vi "CAP-MOD-4.vi"(0 "Count per volt":dbl, 1 "Boolean 3":bool, 2 "Numeric 10":dbl, 3 "data[2]":u8, 4 "data[3]":u8, 5 "data[4]":u8, 6 "data[5]":u8, 8 "Boolean":bool, 9 "data[6]":u8, 10 "Boolean 2":bool, 11 "data[7]":u8, 12 "Numeric 9":dbl, 13 "Numeric 12":dbl, 14 "Numeric 8":dbl, 15 "Numeric 11":dbl, 16 "Numeric 7":dbl) -> (18 "Numeric 4":dbl, 20 "Numeric 5":dbl, 21 "Numeric 6":dbl, 22 "Numeric 3":dbl, 23 "Numeric":dbl, 24 "Numeric 2":dbl)   [LabVIEW 2016]
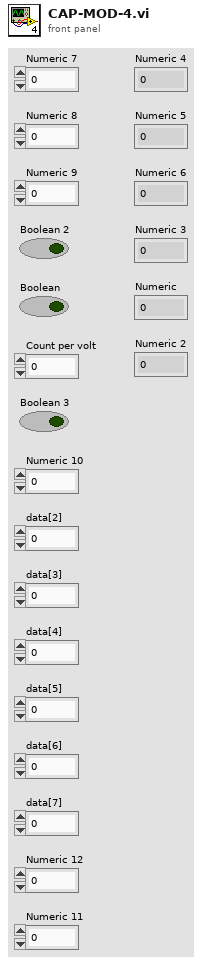
[diagram p1: front panel]
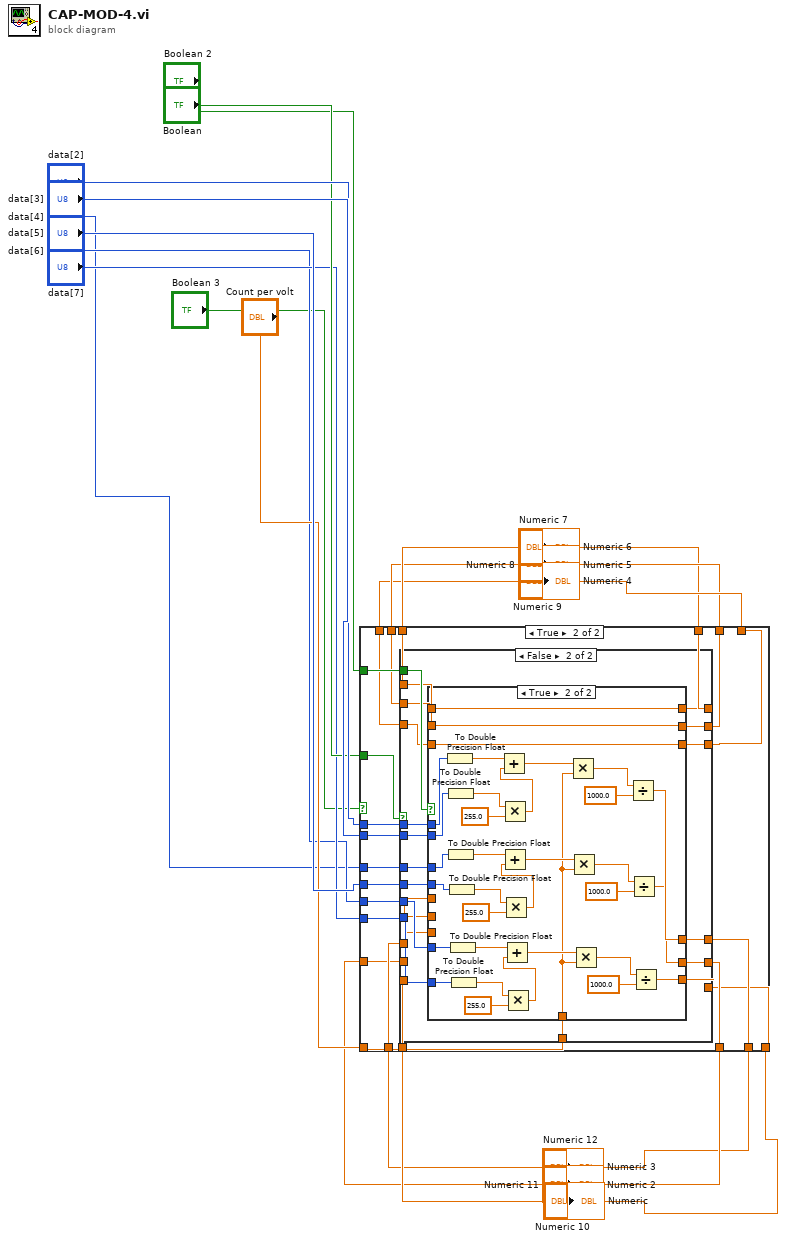
[diagram p0: block diagram]
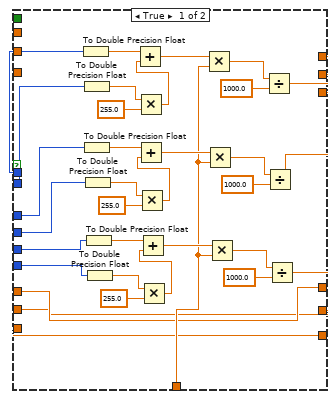
[diagram p3: hidden frame]
diagram:
  n1 = case shown="True" "Boolean 3" {
    tunnel: "Boolean 2" -> [_ w49]
    tunnel: "Boolean" -> [_ w48]
    tunnel: [w23 w47] -> w15
    tunnel: "Numeric 7" -> [w23 w46]
    tunnel: [w24 w45] -> w16
    tunnel: "Numeric 8" -> [w24 w44]
    tunnel: "Numeric 9" -> [w25 w43]
    tunnel: [w25 w42] -> w17
    tunnel: [w28 w41] -> w18
    tunnel: [w27 w40] -> w19
    tunnel: [w26 w39] -> w20
    tunnel: "Numeric 12" -> [w28 w38]
    tunnel: "Numeric 11" -> [w27 w37]
    tunnel: "Numeric 10" -> [w26 w36]
    tunnel: "data[2]" -> [_ w35]
    tunnel: "data[3]" -> [_ w34]
    tunnel: "data[4]" -> [_ w33]
    tunnel: "data[5]" -> [_ w32]
    tunnel: "data[6]" -> [_ w31]
    tunnel: "data[7]" -> [_ w30]
    tunnel: "Count per volt" -> [_ w29]
    frame False {
    }
    frame True {
      n2 = case shown="False" w48 {
        tunnel: w49 -> [_ w103]
        tunnel: w29 -> [w57 w102]
        tunnel: w35 -> [w63 w101]
        tunnel: w34 -> [w62 w100]
        tunnel: w33 -> [w61 w99]
        tunnel: w32 -> [w60 w98]
        tunnel: w31 -> [w59 w97]
        tunnel: w30 -> [w58 w96]
        tunnel: [w53 w95] -> w41
        tunnel: [w52 w94] -> w40
        tunnel: [w51 w93] -> w39
        tunnel: w38 -> [w53 w92]
        tunnel: w37 -> [w52 w91]
        tunnel: w36 -> [w51 w90]
        tunnel: w46 -> [_ w89]
        tunnel: [w56 w88] -> w47
        tunnel: [w55 w87] -> w45
        tunnel: w44 -> [_ w86]
        tunnel: w43 -> [_ w85]
        tunnel: [w54 w84] -> w42
        frame True {
          n3 = To Double Precision Float(number=w63) -> (double precision float=w69:dbl)
          n4 = To Double Precision Float(number=w62) -> (double precision float=w70:dbl)
          n5 = To Double Precision Float(number=w61) -> (double precision float=w76:dbl)
          n6 = To Double Precision Float(number=w60) -> (double precision float=w77:dbl)
          n7 = To Double Precision Float(number=w59) -> (double precision float=w82:dbl)
          n8 = To Double Precision Float(number=w58) -> (double precision float=w83:dbl)
          n9 = Multiply(x=w70, y=255.0) -> (x*y=w67:dbl)
          n10 = Add(x=w69, y=w67) -> (x+y=w65:dbl)
          n11 = Multiply(x=w77, y=255.0) -> (x*y=w74:dbl)
          n12 = Add(x=w76, y=w74) -> (x+y=w72:dbl)
          n13 = Multiply(x=w83, y=255.0) -> (x*y=w81:dbl)
          n14 = Add(x=w82, y=w81) -> (x+y=w79:dbl)
          n15 = Multiply(x=w65, y=w57) -> (x*y=w66:dbl)
          n16 = Multiply(x=w72, y=w57) -> (x*y=w73:dbl)
          n17 = Multiply(x=w79, y=w57) -> (x*y=w80:dbl)
          n18 = Divide(x=w66, y=1000.0) -> (x/y=w56:dbl)
          n19 = Divide(x=w73, y=1000.0) -> (x/y=w55:dbl)
          n20 = Divide(x=w80, y=1000.0) -> (x/y=w54:dbl)
        }
        frame False {
          n21 = case shown="True" w103 {
            tunnel: w102 -> [_ w110]
            tunnel: w101 -> [_ w138]
            tunnel: w100 -> [_ w135]
            tunnel: w99 -> [_ w120]
            tunnel: w98 -> [_ w119]
            tunnel: w97 -> [_ w118]
            tunnel: w96 -> [_ w117]
            tunnel: [w106 w116] -> w95
            tunnel: [w105 w115] -> w94
            tunnel: [w104 w114] -> w93
            tunnel: w92 -> [w106 _]
            tunnel: w91 -> [w105 _]
            tunnel: w90 -> [w104 _]
            tunnel: w89 -> [w109 w113]
            tunnel: [w109 w113] -> w88
            tunnel: [w108 w112] -> w87
            tunnel: w86 -> [w108 w112]
            tunnel: [w107 w111] -> w84
            tunnel: w85 -> [w107 w111]
            frame False {
            }
            frame True {
              n22 = To Double Precision Float(number=w138) -> (double precision float=w137:dbl)
              n23 = To Double Precision Float(number=w135) -> (double precision float=w136:dbl)
              n24 = To Double Precision Float(number=w120) -> (double precision float=w129:dbl)
              n25 = To Double Precision Float(number=w119) -> (double precision float=w128:dbl)
              n26 = To Double Precision Float(number=w118) -> (double precision float=w122:dbl)
              n27 = To Double Precision Float(number=w117) -> (double precision float=w121:dbl)
              n28 = Multiply(x=w136, y=255.0) -> (x*y=w140:dbl)
              n29 = Add(x=w137, y=w140) -> (x+y=w142:dbl)
              n30 = Multiply(x=w128, y=255.0) -> (x*y=w131:dbl)
              n31 = Add(x=w129, y=w131) -> (x+y=w133:dbl)
              n32 = Multiply(x=w121, y=255.0) -> (x*y=w124:dbl)
              n33 = Add(x=w122, y=w124) -> (x+y=w126:dbl)
              n34 = Multiply(x=w142, y=w110) -> (x*y=w141:dbl)
              n35 = Multiply(x=w133, y=w110) -> (x*y=w132:dbl)
              n36 = Multiply(x=w126, y=w110) -> (x*y=w125:dbl)
              n37 = Divide(x=w141, y=1000.0) -> (x/y=w116:dbl)
              n38 = Divide(x=w132, y=1000.0) -> (x/y=w115:dbl)
              n39 = Divide(x=w125, y=1000.0) -> (x/y=w114:dbl)
            }
          }
        }
      }
    }
  }
  "Numeric" <- w20
  "Numeric 2" <- w19
  "Numeric 3" <- w18
  "Numeric 4" <- w17
  "Numeric 5" <- w16
  "Numeric 6" <- w15
